vi "HighEnd-FPGA.vi"() -> ()   [LabVIEW 2016]
uses:
  Aperture Readback.ctl
  Faraday Cup Readback.ctl
  Glassman Readback.ctl
  Glassman Control.ctl
  <vilib>/LabVIEW Targets/FPGA/cRIO/shared/nicrio_ModuleControls/nicrio_cRIO-9871_BaudRateEnum.ctl
  <vilib>/LabVIEW Targets/FPGA/cRIO/shared/nicrio_ModuleControls/nicrio_cRIO-9871_DataBitsEnum.ctl
  <vilib>/LabVIEW Targets/FPGA/cRIO/shared/nicrio_ModuleControls/nicrio_cRIO-9871_ParityEnum.ctl
  <vilib>/LabVIEW Targets/FPGA/cRIO/shared/nicrio_ModuleControls/nicrio_cRIO-9871_StopBitsEnum.ctl
  <vilib>/Platform/TimedLoop/XDataNode/timing_clust.ctl
  <vilib>/Platform/TimedLoop/XDataNode/nitl_modes.ctl
  <vilib>/Platform/TimedLoop/XDataNode/wakeup.ctl
  <vilib>/rvi/FXPMathLib/basic elements/FxpIntAccumulator/subVIs/nifxpmath_IntAccumulator_SimConfig.ctl
  Gate Valve Readback.ctl
  <vilib>/rvi/Emulation/niFpgaGetClockAttributes.vi
  <vilib>/rvi/Emulation/niFpgaSctlEmulationGetInTimedLoop.vi
  <vilib>/rvi/Emulation/niFpgaEmulationReportErrorSimple.vi
  <vilib>/rvi/eio/common/nirviEmuTemplateMethod_errors.vi
  <vilib>/rvi/Emulation/niFpgaCriticalErrorInLSC.vi
  <vilib>/rvi/Analysis/common/codeGenErrors/XNode/niFpgaXNodeCodeGenErrorHandle.vi
  <vilib>/rvi/FXPMathLib/basic elements/FxpIntAccumulator/simVIs/DllFxpIntAccumulator_sub.vi
  <vilib>/rvi/eio/common/nirviEmuTemplatePropertySet_errors.vi
  <vilib>/eio/EIONode/EIONode.xnode
  <vilib>/rvi/Analysis/measure/dc-rms/XNode/niFpgaDC-RMS.xnode
  <vilib>/Platform/TimedLoop/XDataNode/XDataNode.xnode
  <vilib>/rvi/FXPMathLib/basic elements/FxpIntAccumulator/XNode/nifxpmath_IntAccumulator.xnode
  <vilib>/rvi/FXPMathLib/FxpMul/XNode/nifxpmath_Multiplier.xnode
  <vilib>/eio/EIOPropertyNode/EIOPropertyNode.xnode
  <vilib>/eio/EIOMethodNode/EIOMethodNode.xnode
  <vilib>/Platform/TimedLoop/XDataNode/XDNodeRunTimeDep.lvlib
  <vilib>/rvi/FXPMathLib/sim/FxpSim.dll
  <vilib>/rvi/eio/common/nirviEmuTemplatePropertyGet_errors.vi
  <vilib>/rvi/eio/common/nirviEmuTemplatePropertyGet_noerrors.vi
  <vilib>/rvi/eio/common/nirviEmuTemplatePropertySet_noerrors.vi
panel:
  out "HV control loop error":errorcluster
  in  "ES Quad A V set":T1
  in  "Y1- Steerer V set":T1
  in  "ES Quad B V set":T1
  in  "Y2- Steerer V set":T1
  in  "Y2+ Steerer V set":T1
  in  "Y1+ Steerer V set":T1
  in  "X- Steerer V set":T1
  in  "X+ Steerer V set":T1
  out "ES Quad HV readback loop error":errorcluster
  out "ES Quad B- readback":T2
  out "ES Quad B+ readback":T2
  out "ES Quad A- readback":T2
  out "ES Quad A+ readback":T2
  out "Steerer HV readback loop error":errorcluster
  out "Y2- Steerer readback":T2
  out "Y2+ Steerer readback":T2
  out "Y1- Steerer readback":T2
  out "Y1+ Steerer readback":T2
  out "X- Steerer readback":T2
  out "X+ Steerer readback":T2
  out "Analyzer Object Ion Gauge 2":u8[](array[numeric])
  out "Analyzer Object Convectron 2":u8[](array[numeric])
  out "Analyzer Object Convectron 1":u8[](array[numeric])
  out "Analyzer Object Ion Gauge 1":u8[](array[numeric])
  out "Analyzer Obj Vac Gauge error":errorcluster
  out "Tank Exit Ion Gauge 2":u8[](array[numeric])
  out "Tank Exit Convectron 2":u8[](array[numeric])
  out "Tank Exit Convectron 1":u8[](array[numeric])
  out "Tank Exit Ion Gauge 1":u8[](array[numeric])
  out "Tank Exit Vac Gauge error":errorcluster
  out "Beamline Fast GV Position":T3
  in  "Tank Exit FC Actuator":bool
  out "Tank Exit FC Position":T4
  out "Beamline GV Position":T4
  out "Cryo Pump GV Position":T3
  out "Turbo GV Position":T3
  out "Actuator loop error":errorcluster
  in  "Beamline GV Actuator":bool
  in  "Cryo Pump GV Actuator":bool
  in  "Turbo GV actuator":bool
  in  "Beamline Fast GV actuator":bool
  out "Tank Exit Vac Interlock":bool
  out "High End Waist Vac Interlock":bool
  in  "Analyzer Image Vac Interlock":bool
  in  "Tank Exit interlock bypass":bool
  in  "High End waist interlock bypass":bool
  out "GV Interlock loop error 2":errorcluster
  in  "RT error":bool
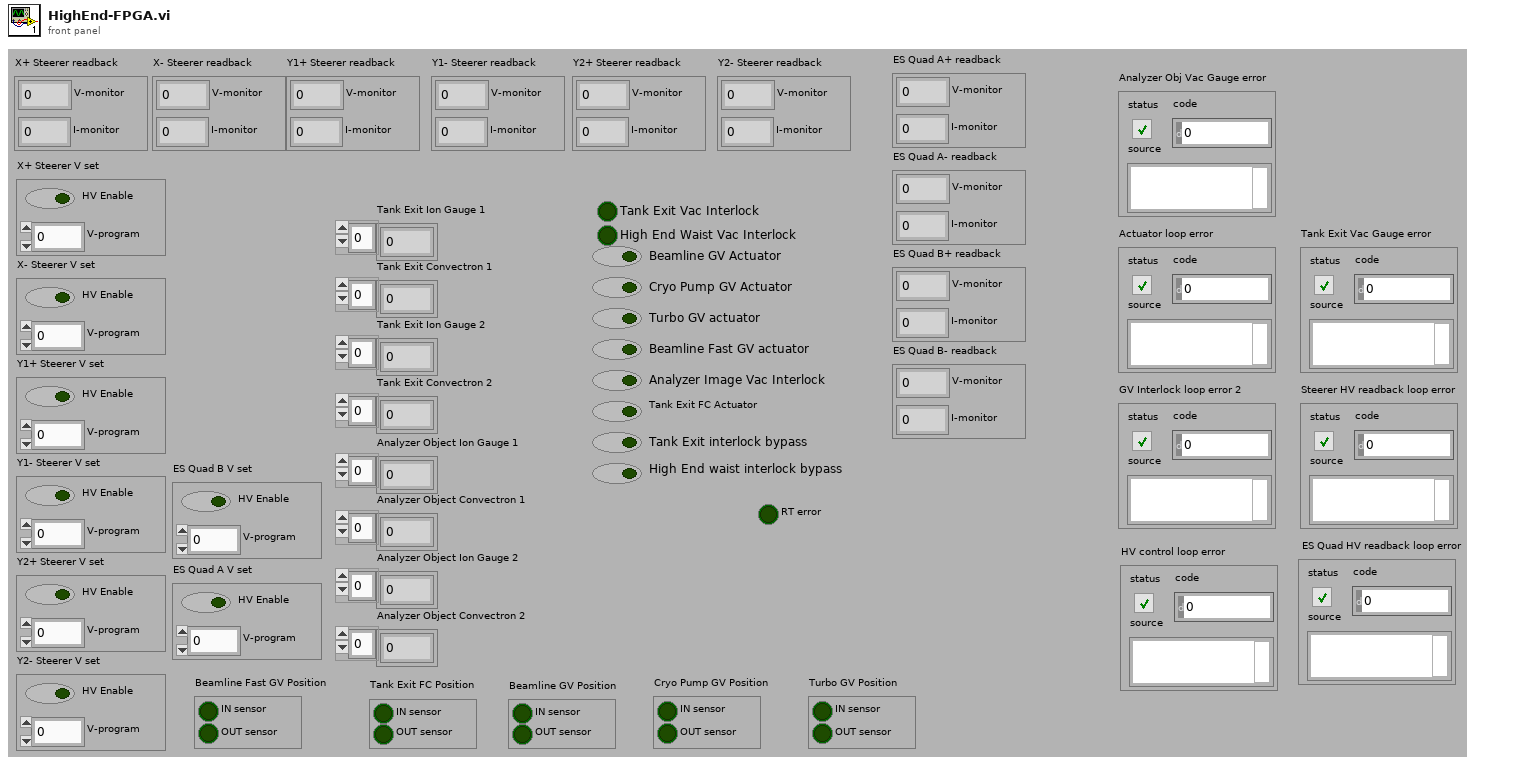
[diagram p1: front panel]
types:
  T1 = typedef "Glassman Control.ctl" = cluster{"V-program":fxp<+/-,20,5>, "HV Enable":bool}
  T2 = typedef "Glassman Readback.ctl" = cluster{"I-monitor":fxp<+/-,26,5>, "V-monitor":fxp<+/-,26,7>}
  T3 = typedef "Aperture Readback.ctl" = cluster{"IN sensor":bool, "OUT sensor":bool}
  T4 = typedef "Faraday Cup Readback.ctl" = cluster{"IN sensor":bool, "OUT sensor":bool}
  T5 = typedef "nicrio_cRIO-9871_StopBitsEnum.ctl" = enum8{"1", "1.5", "2"}
  T6 = typedef "nicrio_cRIO-9871_ParityEnum.ctl" = enum8{"None", "Odd", "Even", "Mark", "Space"}
  T7 = typedef "nicrio_cRIO-9871_DataBitsEnum.ctl" = enum8{"5", "6", "7", "8"}
  T8 = typedef "nicrio_cRIO-9871_BaudRateEnum.ctl" = enum16{"75 bps", "110 bps", "134 bps", "150 bps", "300 bps", "600 bps", "1200 bps", "1800 bps", "2400 bps", "4800 bps", "7200 bps", "9600 bps", "14.4 kbps", "19.2 kbps", "28.8 kbps", "38.4 kbps", "57.6 kbps", "115.2 kbps", "230.4 kbps", "460.8 kbps", "921.6 kbps"}
  T9 = typedef "Gate Valve Readback.ctl" = cluster{"OPEN sensor":bool, "Closed sensor":bool}
  T10 = typedef "XDNodeRunTimeDep.lvlib/timing_clust.ctl" = cluster{"Expected End [f-1]":u64, "Actual End [f-1]":u64, "Finished Late? [f-1]":bool, "Expected End [i-1]":u64, "Actual End [i-1]":u64, "Finished Late? [i-1]":bool, "Expected Start [i]":u64, "Actual Start [i]":u64, "Expected Start [f]":u64, "Actual Start [f]":u64, "Source Name":string, "Structure Name":string, "Period":i64, "Deadline":i64, "Offset":i64, "Start":i64, "Priority":i32, "Timeout":i32, "Mode":T11, "Wakeup Reason":T12, "Error":errorcluster, "Source Type":string, "Secondary Source Type":string, "Global End Time":u64, "Global Start Time":u64, "Frame Duration":u64, "Iteration Duration":u64, "Assigned CPU":i32, "I/O Scan Engine Mode":u32}
  T11 = typedef "XDNodeRunTimeDep.lvlib/nitl_modes.ctl" = enum32{"No Change", "Process missed periods, maintain original phase", "Discard missed periods, maintain original phase", "Process missed periods, ignore original phase", "Discard missed periods, ignore original phase"}
  T12 = typedef "XDNodeRunTimeDep.lvlib/wakeup.ctl" = enum32{"Normal", "Aborted", "Asynchronous wakeup", "Timing source error", "Timed loop error", "Timeout"}
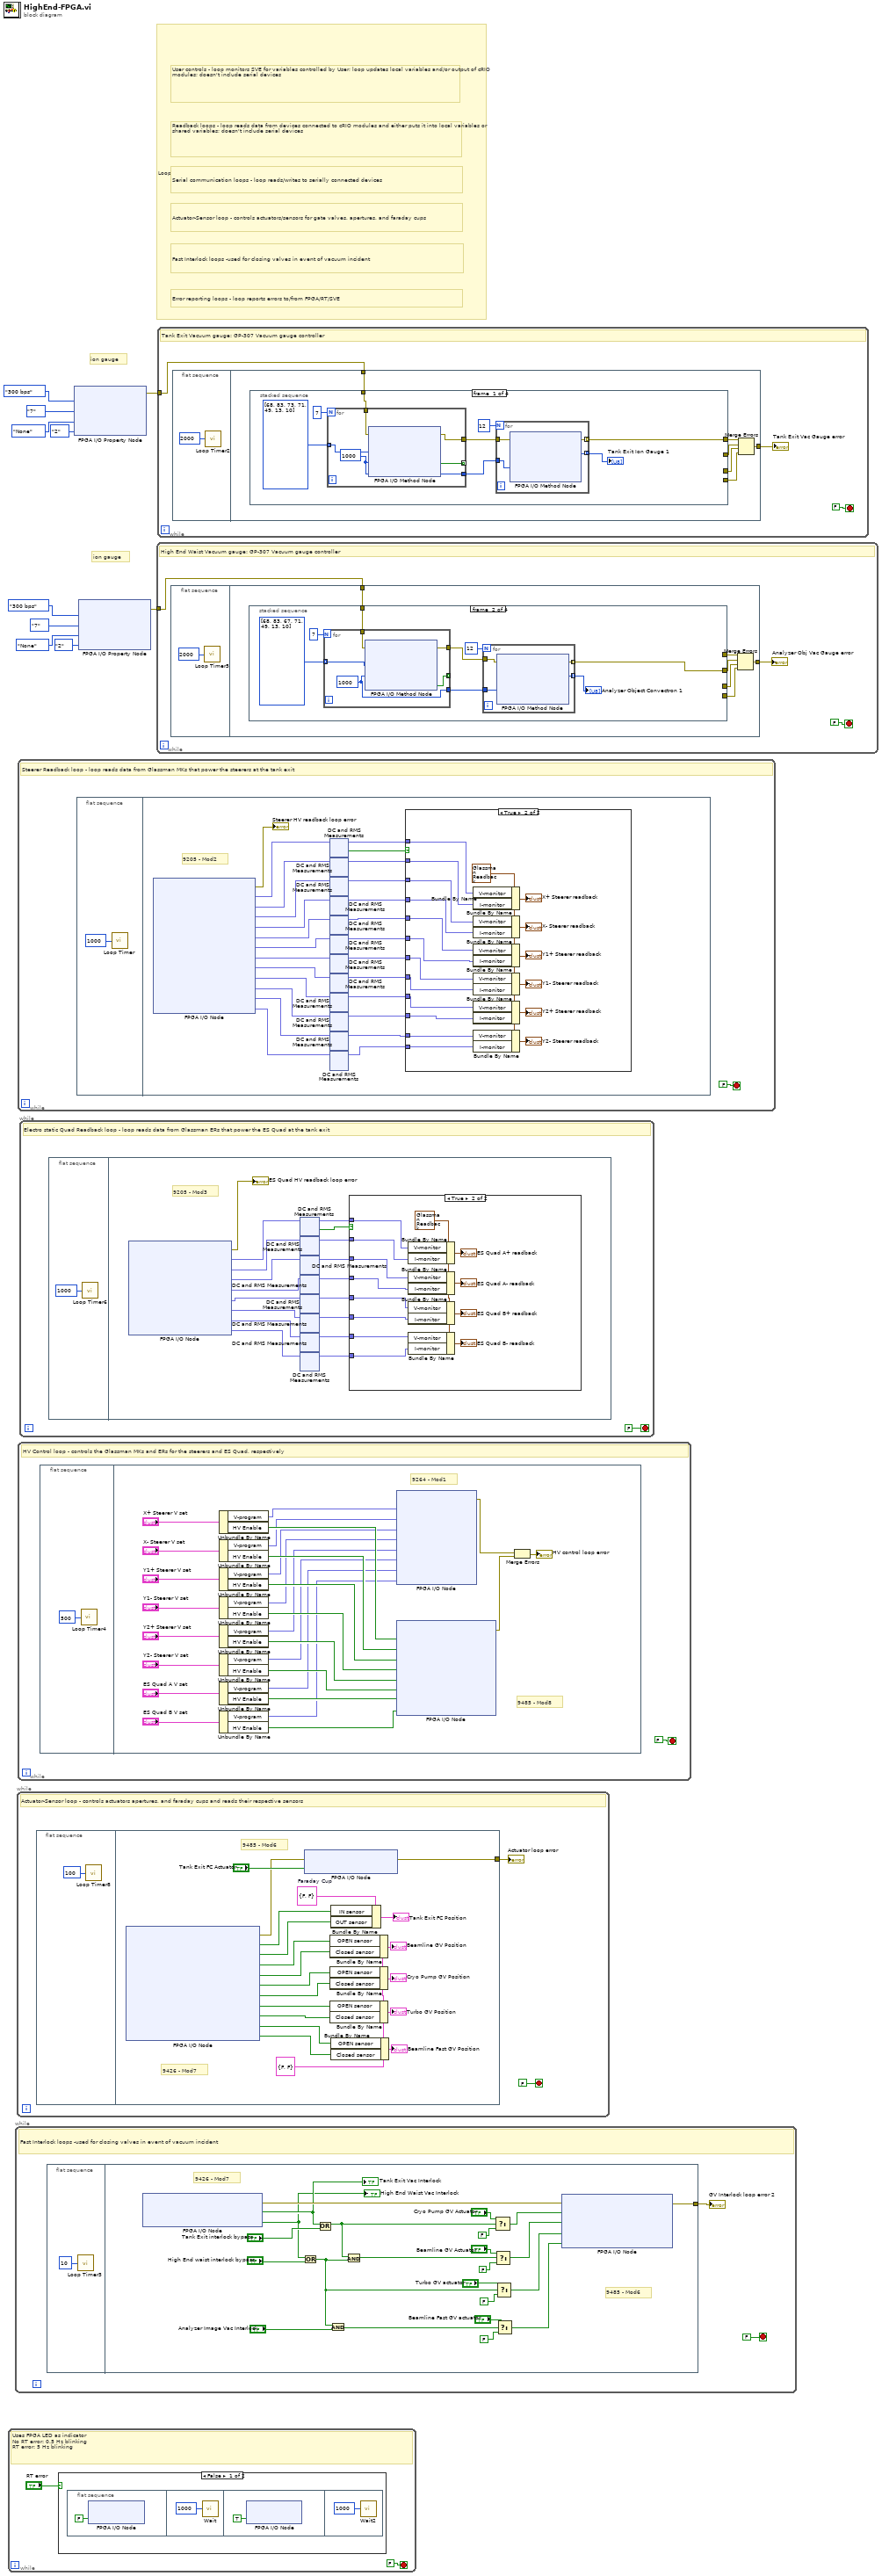
[diagram p0: block diagram]
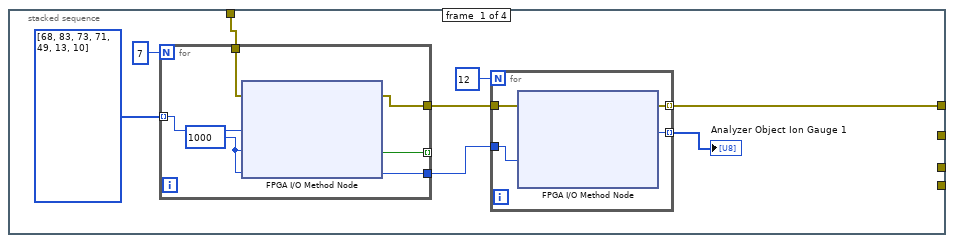
[diagram p3: hidden frame]
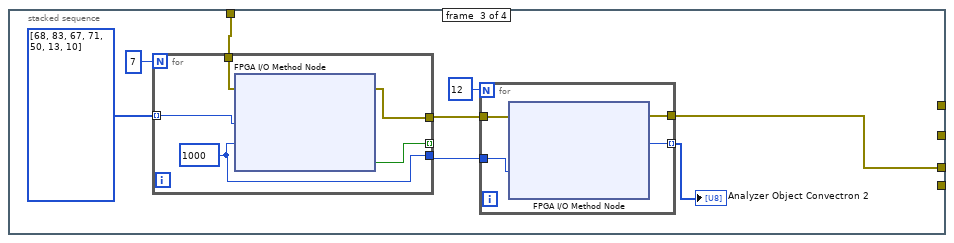
[diagram p4: hidden frame]
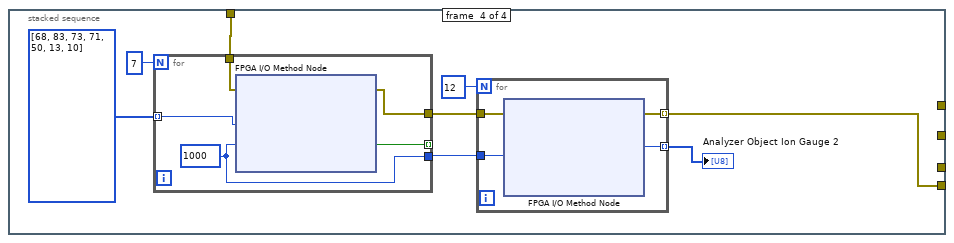
[diagram p5: hidden frame]
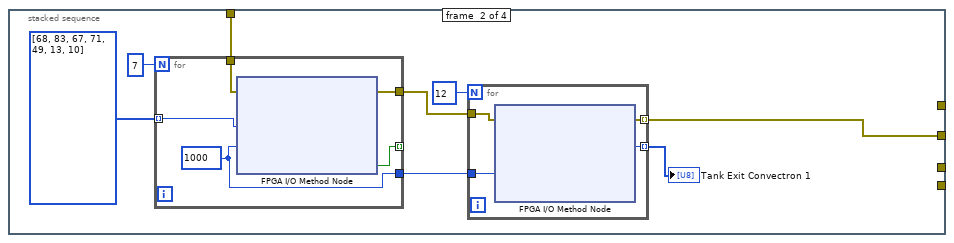
[diagram p6: hidden frame]
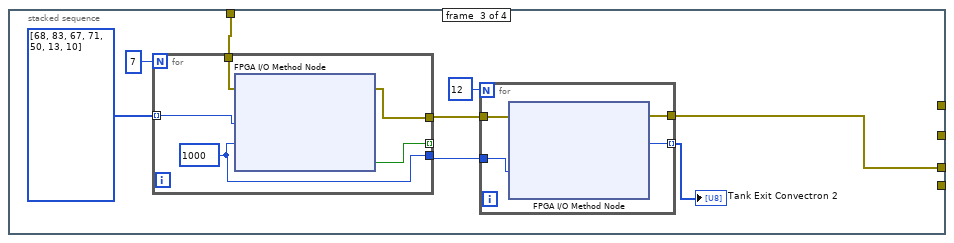
[diagram p7: hidden frame]
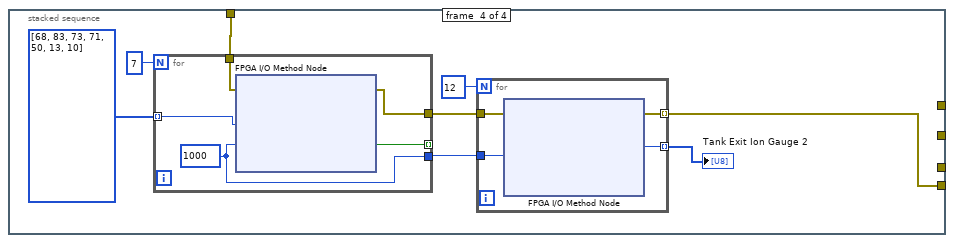
[diagram p8: hidden frame]
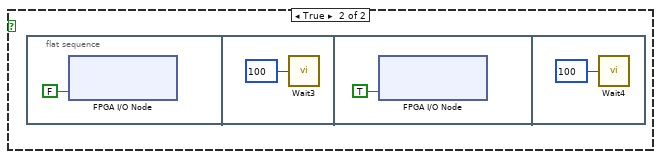
[diagram p9: hidden frame]
diagram:
  # "ion gauge"
  # "ion gauge"
  # "Actuator-Sensor loop - controls actuators/sensors for gate valves, apertures, and faraday cups"
  # "Fast Interlock loops -used for closing valves in event of vacuum incident"
  # "Error reporting loops - loop reports errors to/from FPGA/RT/SVE"
  # "Serial communication loops - loop reads/writes to serially connected devices"
  # "Readback loops - loop reads data from devices connected to cRIO modules and either puts it into local variables or shared variables; doesn't include serial devices"
  # "User controls - loop monitors SVE for variables controlled by User; loop updates local variables and/or output of cRIO modules; doesn't include serial devices"
  # "Loop legend - loops are color coded by responsibility"
  n1 = while {
    stop <- FALSE stop-if-true
    # "Uses FPGA LED as indicator\nNo RT error: 0.5 Hz blinking\nRT error: 5 Hz blinking"
    n2 = case shown="False" "RT error" {
      frame False {
        n3 = flat-sequence {
          frame #0 {
            n4 = xnode "FPGA I/O Node"("FPGA LED"=FALSE) -> ()  [unwired: 1 in, 1 out]
          }
          frame #1 {
            n5 = call "Wait"("Count(mSec)"=u16 1000) -> ()  [unwired: 1 out]
          }
          frame #2 {
            n6 = xnode "FPGA I/O Node"("FPGA LED"=TRUE) -> ()  [unwired: 1 in, 1 out]
          }
          frame #3 {
            n7 = call "Wait2"("Count(mSec)"=u16 1000) -> ()  [unwired: 1 out]
          }
        }
      }
      frame True {
        n8 = flat-sequence {
          frame #0 {
            n9 = xnode "FPGA I/O Node"("FPGA LED"=FALSE) -> ()  [unwired: 1 in, 1 out]
          }
          frame #1 {
            n10 = call "Wait3"("Count(mSec)"=u16 100) -> ()  [unwired: 1 out]
          }
          frame #2 {
            n11 = xnode "FPGA I/O Node"("FPGA LED"=TRUE) -> ()  [unwired: 1 in, 1 out]
          }
          frame #3 {
            n12 = call "Wait4"("Count(mSec)"=u16 100) -> ()  [unwired: 1 out]
          }
        }
      }
    }
  }
  n13 = while {
    stop <- FALSE stop-if-true
    # "Fast Interlock loops -used for closing valves in event of vacuum incident"
    n14 = flat-sequence {
      tunnel: [w35] -> w21
      frame #0 {
        n15 = call "Loop Timer3"("Count(uSec)"=u32 10) -> ()  [unwired: 1 out]
      }
      frame #1 {
        # "9485 - Mod6"
        # "9426 - Mod7"
        n16 = xnode "FPGA I/O Node"() -> ("error out"=w46:errorcluster, "Tank Exit Vac Interlock"=w34:bool, "High End Waist Vac Interlock"=w32:bool)  [unwired: 3 in, 2 out]
        "Tank Exit Vac Interlock" <- w34
        "High End Waist Vac Interlock" <- w32
        n17 = Or(x=w32, y="High End waist interlock bypass") -> (x .or. y?=w25:bool)
        n18 = Or(x=w34, y="Tank Exit interlock bypass") -> (x .or. y?=w24:bool)
        n19 = And(x=w25, y="Analyzer Image Vac Interlock") -> (x .and. y?=w30:bool)
        n20 = And(x=w24, y=w25) -> (x .and. y?=w26:bool)
        n21 = Select(t="Cryo Pump GV Actuator", s=w24, f=FALSE) -> (s? t:f=w36:bool)
        n22 = Select(t="Beamline GV Actuator", s=w26, f=FALSE) -> (s? t:f=w38:bool)
        n23 = Select(t="Turbo GV actuator", s=w25, f=FALSE) -> (s? t:f=w41:bool)
        n24 = Select(t="Beamline Fast GV actuator", s=w30, f=FALSE) -> (s? t:f=w44:bool)
        n25 = xnode "FPGA I/O Node"("error in"=w46, "Cryo Pump GV actuator"=w36, "Beamline GV actuator"=w38, "Turbo GV actuator"=w41, "Beamline Fast GV actuator"=w44) -> ("error out"=w35:errorcluster)  [unwired: 4 in, 4 out]
      }
    }
    "GV Interlock loop error 2" <- w21
  }
  n26 = while {
    stop <- FALSE stop-if-true
    # "Actuator-Sensor loop - controls actuators apertures, and faraday cups and reads their respective sensors"
    n27 = flat-sequence {
      tunnel: [w68] -> w47
      frame #0 {
        n28 = call "Loop Timer8"("Count(mSec)"=u32 100 ("Count(uSec)")) -> ()  [unwired: 1 out]
      }
      frame #1 {
        w52 = T9 {"OPEN sensor"=FALSE, "Closed sensor"=FALSE} ("Gate Valve")
        w64 = T4 {"IN sensor"=FALSE, "OUT sensor"=FALSE}  # Faraday Cup
        # "9485 - Mod6"
        # "9426 - Mod7"
        n29 = xnode "FPGA I/O Node"() -> ("error out"=w67:errorcluster, "Tank Exit FC IN sensor"=w66:bool, "Tank Exit FC OUT sensor"=w65:bool, "Beamline GV OPEN sensor"=w59:bool, "Beamline GV CLOSED sensor"=w58:bool, "Cryo Pump GV OPEN sensor"=w57:bool, "Cryo Pump GV CLOSED sensor"=w56:bool, "Turbo GV OPEN sensor"=w55:bool, "Turbo GV CLOSED sensor"=w54:bool, "Beamline Fast GV OPEN sensor"=w51:bool, "Beamline Fast GV CLOSED sensor"=w50:bool)  [unwired: 11 in, 10 out]
        n30 = xnode "FPGA I/O Node"("error in"=w67, "Tank Exit FC actuator"="Tank Exit FC Actuator") -> ("error out"=w68:errorcluster)  [unwired: 1 in, 1 out]
        n31 = Bundle By Name(cluster=w52, "OPEN sensor"=w59, "Closed sensor"=w58) -> (→"Beamline GV Position":T9)
        n32 = Bundle By Name(cluster=w52, "OPEN sensor"=w57, "Closed sensor"=w56) -> (→"Cryo Pump GV Position":T9)
        n33 = Bundle By Name(cluster=w52, "OPEN sensor"=w55, "Closed sensor"=w54) -> (→"Turbo GV Position":T9)
        n34 = Bundle By Name(cluster=w64, "IN sensor"=w66, "OUT sensor"=w65) -> (→"Tank Exit FC Position":T4)
        n35 = Bundle By Name(cluster=w52, "OPEN sensor"=w51, "Closed sensor"=w50) -> (→"Beamline Fast GV Position":T9)
      }
    }
    "Actuator loop error" <- w47
  }
  n36 = while {
    stop <- FALSE stop-if-true
    # "Steerer Readback loop - loop reads data from Glassman MKs that power the steerers at the tank exit"
    n37 = flat-sequence {
      frame #0 {
        n38 = call "Loop Timer"("Count(Ticks)"=u32 1000) -> ()  [unwired: 1 out]
      }
      frame #1 {
        # "9205 - Mod2"
        n39 = xnode "FPGA I/O Node"() -> ("error out"=→"Steerer HV readback loop error":errorcluster, "X+ Steerer V readback"=w96:fxp<+/-,26,5>, "X+ Steerer I readback"=w94:fxp<+/-,26,5>, "X- Steerer V readback"=w92:fxp<+/-,26,5>, "X- Steerer I readback"=w90:fxp<+/-,26,5>, "Y1+ Steerer V readback"=w88:fxp<+/-,26,5>, "Y1+ Steerer I readback"=w86:fxp<+/-,26,5>, "Y1- Steerer V readback"=w84:fxp<+/-,26,5>, "Y1- Steerer I readback"=w82:fxp<+/-,26,5>, "Y2+ Steerer V readback"=w80:fxp<+/-,26,5>, "Y2+ Steerer I readback"=w78:fxp<+/-,26,5>, "Y2- Steerer V readback"=w76:fxp<+/-,26,5>, "Y2- Steerer I readback"=w73:fxp<+/-,26,5>)  [unwired: 13 in, 12 out]
        n40 = xnode "DC and RMS Measurements"("input data"=w96) -> ("DC"=w95:fxp<+/-,26,5>, "output valid"=w97:bool)  [unwired: 1 in]
        n41 = xnode "DC and RMS Measurements"("input data"=w94) -> ("DC"=w93:fxp<+/-,26,5>)  [unwired: 1 in, 1 out]
        n42 = xnode "DC and RMS Measurements"("input data"=w92) -> ("DC"=w91:fxp<+/-,26,5>)  [unwired: 1 in, 1 out]
        n43 = xnode "DC and RMS Measurements"("input data"=w90) -> ("DC"=w89:fxp<+/-,26,5>)  [unwired: 1 in, 1 out]
        n44 = xnode "DC and RMS Measurements"("input data"=w88) -> ("DC"=w87:fxp<+/-,26,5>)  [unwired: 1 in, 1 out]
        n45 = xnode "DC and RMS Measurements"("input data"=w86) -> ("DC"=w85:fxp<+/-,26,5>)  [unwired: 1 in, 1 out]
        n46 = xnode "DC and RMS Measurements"("input data"=w84) -> ("DC"=w83:fxp<+/-,26,5>)  [unwired: 1 in, 1 out]
        n47 = xnode "DC and RMS Measurements"("input data"=w82) -> ("DC"=w81:fxp<+/-,26,5>)  [unwired: 1 in, 1 out]
        n48 = xnode "DC and RMS Measurements"("input data"=w80) -> ("DC"=w79:fxp<+/-,26,5>)  [unwired: 1 in, 1 out]
        n49 = xnode "DC and RMS Measurements"("input data"=w78) -> ("DC"=w77:fxp<+/-,26,5>)  [unwired: 1 in, 1 out]
        n50 = xnode "DC and RMS Measurements"("input data"=w76) -> ("DC"=w75:fxp<+/-,26,5>)  [unwired: 1 in, 1 out]
        n51 = xnode "DC and RMS Measurements"("input data"=w73) -> ("DC"=w74:fxp<+/-,26,5>)  [unwired: 1 in, 1 out]
        n52 = case shown="True" w97 {
          tunnel: w95 -> [_ w196]
          tunnel: w93 -> [_ w195]
          tunnel: w91 -> [_ w194]
          tunnel: w89 -> [_ w193]
          tunnel: w87 -> [_ w192]
          tunnel: w85 -> [_ w191]
          tunnel: w83 -> [_ w190]
          tunnel: w81 -> [_ w189]
          tunnel: w79 -> [_ w188]
          tunnel: w77 -> [_ w187]
          tunnel: w75 -> [_ w186]
          tunnel: w74 -> [_ w185]
          frame False {
          }
          frame True {
            w178 = T2 {"I-monitor"=0.0, "V-monitor"=0.0} ("Glassman Readback")
            n53 = Bundle By Name(cluster=w178, "V-monitor"=w196, "I-monitor"=w195) -> (→"X+ Steerer readback":T2)
            n54 = Bundle By Name(cluster=w178, "V-monitor"=w194, "I-monitor"=w193) -> (→"X- Steerer readback":T2)
            n55 = Bundle By Name(cluster=w178, "V-monitor"=w192, "I-monitor"=w191) -> (→"Y1+ Steerer readback":T2)
            n56 = Bundle By Name(cluster=w178, "V-monitor"=w190, "I-monitor"=w189) -> (→"Y1- Steerer readback":T2)
            n57 = Bundle By Name(cluster=w178, "V-monitor"=w188, "I-monitor"=w187) -> (→"Y2+ Steerer readback":T2)
            n58 = Bundle By Name(cluster=w178, "V-monitor"=w186, "I-monitor"=w185) -> (→"Y2- Steerer readback":T2)
          }
        }
      }
    }
  }
  n59 = while {
    stop <- FALSE stop-if-true
    # "HV Control loop - controls the Glassman MKs and ERs for the steerers and ES Quad, respectively"
    n60 = flat-sequence {
      frame #0 {
        n61 = call "Loop Timer4"("Count(uSec)"=u32 500 ("Count(Ticks)")) -> ()  [unwired: 1 out]
      }
      frame #1 {
        # "9485 - Mod8"
        # "9264 - Mod1"
        n62 = Unbundle By Name("X+ Steerer V set") -> ("V-program"=w1082:fxp<+/-,20,5>, "HV Enable"=w1090:bool)
        n63 = Unbundle By Name("X- Steerer V set") -> ("V-program"=w1083:fxp<+/-,20,5>, "HV Enable"=w1091:bool)
        n64 = Unbundle By Name("Y1+ Steerer V set") -> ("V-program"=w1084:fxp<+/-,20,5>, "HV Enable"=w1092:bool)
        n65 = Unbundle By Name("Y1- Steerer V set") -> ("V-program"=w1085:fxp<+/-,20,5>, "HV Enable"=w1093:bool)
        n66 = Unbundle By Name("Y2+ Steerer V set") -> ("V-program"=w1086:fxp<+/-,20,5>, "HV Enable"=w1094:bool)
        n67 = Unbundle By Name("Y2- Steerer V set") -> ("V-program"=w1087:fxp<+/-,20,5>, "HV Enable"=w1095:bool)
        n68 = Unbundle By Name("ES Quad A V set") -> ("V-program"=w1088:fxp<+/-,20,5>, "HV Enable"=w1096:bool)
        n69 = Unbundle By Name("ES Quad B V set") -> ("V-program"=w1089:fxp<+/-,20,5>, "HV Enable"=w1097:bool)
        n70 = xnode "FPGA I/O Node"("X+ Steerer V set"=w1082, "X- Steerer V set"=w1083, "Y1+ Steerer V set"=w1084, "Y1- Steerer V set"=w1085, "Y2+ Steerer V set"=w1086, "Y2- Steerer V set"=w1087, "ES Quad A V set"=w1088, "ES Quad B V set"=w1089) -> ("error out"=w1081:errorcluster)  [unwired: 9 in, 8 out]
        n71 = xnode "FPGA I/O Node"("X+ Steerer HV Enable"=w1090, "X- Steerer HV Enable"=w1091, "Y1+ Steerer HV Enable"=w1092, "Y1- Steerer HV Enable"=w1093, "Y2+ Steerer HV Enable"=w1094, "Y2- Steerer HV Enable"=w1095, "ES Quad A HV Enable"=w1096, "ES Quad B HV Enable"=w1097) -> ("error out"=w1080:errorcluster)  [unwired: 9 in, 8 out]
        n72 = Merge Errors(w1081, w1080) -> (→"HV control loop error":errorcluster)
      }
    }
  }
  n73 = while {
    stop <- FALSE stop-if-true
    # "Electro static Quad Readback loop - loop reads data from Glassman ERs that power the ES Quad at the tank exit"
    n74 = flat-sequence {
      frame #0 {
        n75 = call "Loop Timer6"("Count(Ticks)"=u32 1000) -> ()  [unwired: 1 out]
      }
      frame #1 {
        # "9205 - Mod3"
        n76 = xnode "FPGA I/O Node"() -> ("error out"=→"ES Quad HV readback loop error":errorcluster, "ES Quad A+ V readback"=w1117:fxp<+/-,26,5>, "ES Quad A+ I readback"=w1116:fxp<+/-,26,5>, "ES Quad A- V readback"=w1115:fxp<+/-,26,5>, "ES Quad A- I readback"=w1114:fxp<+/-,26,5>, "ES Quad B+ V readback"=w1113:fxp<+/-,26,5>, "ES Quad B+ I readback"=w1112:fxp<+/-,26,5>, "ES Quad B- V readback"=w1111:fxp<+/-,26,5>, "ES Quad B- I readback"=w1110:fxp<+/-,26,5>)  [unwired: 9 in, 8 out]
        n77 = xnode "DC and RMS Measurements"("input data"=w1117) -> ("DC"=w1125:fxp<+/-,26,5>, "output valid"=w1109:bool)  [unwired: 1 in]
        n78 = xnode "DC and RMS Measurements"("input data"=w1116) -> ("DC"=w1124:fxp<+/-,26,5>)  [unwired: 1 in, 1 out]
        n79 = xnode "DC and RMS Measurements"("input data"=w1115) -> ("DC"=w1123:fxp<+/-,26,5>)  [unwired: 1 in, 1 out]
        n80 = xnode "DC and RMS Measurements"("input data"=w1114) -> ("DC"=w1122:fxp<+/-,26,5>)  [unwired: 1 in, 1 out]
        n81 = xnode "DC and RMS Measurements"("input data"=w1113) -> ("DC"=w1121:fxp<+/-,26,5>)  [unwired: 1 in, 1 out]
        n82 = xnode "DC and RMS Measurements"("input data"=w1112) -> ("DC"=w1120:fxp<+/-,26,5>)  [unwired: 1 in, 1 out]
        n83 = xnode "DC and RMS Measurements"("input data"=w1111) -> ("DC"=w1119:fxp<+/-,26,5>)  [unwired: 1 in, 1 out]
        n84 = xnode "DC and RMS Measurements"("input data"=w1110) -> ("DC"=w1118:fxp<+/-,26,5>)  [unwired: 1 in, 1 out]
        n85 = case shown="True" w1109 {
          tunnel: w1125 -> [_ w1138]
          tunnel: w1124 -> [_ w1137]
          tunnel: w1123 -> [_ w1136]
          tunnel: w1122 -> [_ w1135]
          tunnel: w1121 -> [_ w1134]
          tunnel: w1120 -> [_ w1133]
          tunnel: w1119 -> [_ w1132]
          tunnel: w1118 -> [_ w1131]
          frame False {
          }
          frame True {
            w1130 = T2 {"I-monitor"=0.0, "V-monitor"=0.0} ("Glassman Readback")
            n86 = Bundle By Name(cluster=w1130, "V-monitor"=w1138, "I-monitor"=w1137) -> (→"ES Quad A+ readback":T2)
            n87 = Bundle By Name(cluster=w1130, "V-monitor"=w1136, "I-monitor"=w1135) -> (→"ES Quad A- readback":T2)
            n88 = Bundle By Name(cluster=w1130, "V-monitor"=w1134, "I-monitor"=w1133) -> (→"ES Quad B+ readback":T2)
            n89 = Bundle By Name(cluster=w1130, "V-monitor"=w1132, "I-monitor"=w1131) -> (→"ES Quad B- readback":T2)
          }
        }
      }
    }
  }
  n90 = xnode "FPGA I/O Property Node"("Baud Rate"=nicrio_cRIO-9871_BaudRateEnum."300 bps", "Data Bits"=nicrio_cRIO-9871_DataBitsEnum."7", "Parity"=nicrio_cRIO-9871_ParityEnum."None", "Stop Bits"=nicrio_cRIO-9871_StopBitsEnum."2") -> ("error out"=w2:errorcluster)  [unwired: 2 in, 1 out]
  n91 = xnode "FPGA I/O Property Node"("Baud Rate"=nicrio_cRIO-9871_BaudRateEnum."300 bps", "Data Bits"=nicrio_cRIO-9871_DataBitsEnum."7", "Parity"=nicrio_cRIO-9871_ParityEnum."None", "Stop Bits"=nicrio_cRIO-9871_StopBitsEnum."2") -> ("error out"=w1:errorcluster)  [unwired: 2 in, 1 out]
  n92 = while {
    tunnel: w1 -> [w1780]
    stop <- FALSE stop-if-true
    # "High End Waist Vacuum gauge: GP-307 Vacuum gauge controller"
    n93 = flat-sequence {
      tunnel: w1780 -> [w1788]
      tunnel: [w1783] -> w1779
      frame #0 {
        n94 = call "Loop Timer5"("Count(mSec)"=u32 2000 ("Count(Ticks)")) -> ()  [unwired: 1 out]
      }
      frame #1 {
        n95 = stacked-sequence {
          tunnel: [_ _ w1825 _] -> w1785
          tunnel: [_ _ _ w1841] -> w1784
          tunnel: w1788 -> [w1791 w1808 w1823 w1840]
          tunnel: [w1789 _ _ _] -> w1787
          tunnel: [_ w1807 _ _] -> w1786
          frame #0 {
            n96 = for {
              N: 7 -> [_]
              tunnel: [w1805] -> w1792
              tunnel: [w1804] -> _ mode=indexing
              tunnel: u8[] [68, 83, 73, 71, 49, 13, 10] ("unsigned byte array") -> [w1803] mode=indexing
              tunnel: w1791 -> [w1802]
              tunnel: [w1801] -> w1790
              w1805 = 1000 ("Timeout (ms)")
              n97 = xnode "FPGA I/O Method Node"("error in"=w1802, "Data"=w1803, "Timeout (ms)"=w1805) -> ("error out"=w1801:errorcluster, "Timed Out"=w1804:bool)  [unwired: 1 in, 1 out]
            }
            n98 = for {
              N: 12 -> [_]
              tunnel: w1792 -> [w1800]
              tunnel: [w1799] -> w1793 mode=indexing
              tunnel: w1790 -> [w1798]
              tunnel: [w1797] -> w1789 mode=indexing
              n99 = xnode "FPGA I/O Method Node"("error in"=w1798, "Timeout (ms)"=w1800) -> ("error out"=w1797:errorcluster, "Data"=w1799:u8)  [unwired: 1 in, 2 out]
            }
            "Analyzer Object Ion Gauge 1" <- w1793
          }
          frame #1 {
            n100 = for {
              N: 7 -> [_]
              tunnel: [w1821] -> w1813
              tunnel: [w1820] -> _ mode=indexing
              tunnel: u8[] [68, 83, 67, 71, 49, 13, 10] ("unsigned byte array") -> [w1822] mode=indexing
              tunnel: w1808 -> [w1819]
              tunnel: [w1818] -> w1806
              w1821 = 1000 ("Timeout (ms)")
              n101 = xnode "FPGA I/O Method Node"("error in"=w1819, "Data"=w1822, "Timeout (ms)"=w1821) -> ("error out"=w1818:errorcluster, "Timed Out"=w1820:bool)  [unwired: 1 in, 1 out]
            }
            n102 = for {
              N: 12 -> [_]
              tunnel: w1813 -> [w1817]
              tunnel: [w1816] -> w1809 mode=indexing
              tunnel: w1806 -> [w1815]
              tunnel: [w1814] -> w1807 mode=indexing
              n103 = xnode "FPGA I/O Method Node"("error in"=w1815, "Timeout (ms)"=w1817) -> ("error out"=w1814:errorcluster, "Data"=w1816:u8)  [unwired: 1 in, 2 out]
            }
            "Analyzer Object Convectron 1" <- w1809
          }
          frame #2 {
            n104 = for {
              N: 7 -> [_]
              tunnel: [w1837] -> w1830
              tunnel: [w1838] -> _ mode=indexing
              tunnel: u8[] [68, 83, 67, 71, 50, 13, 10] ("unsigned byte array") -> [w1839] mode=indexing
              tunnel: [w1836] -> w1826
              tunnel: w1823 -> [w1835]
              w1837 = 1000 ("Timeout (ms)")
              n105 = xnode "FPGA I/O Method Node"("error in"=w1835, "Data"=w1839, "Timeout (ms)"=w1837) -> ("error out"=w1836:errorcluster, "Timed Out"=w1838:bool)  [unwired: 1 in, 1 out]
            }
            n106 = for {
              N: 12 -> [_]
              tunnel: w1830 -> [w1834]
              tunnel: [w1833] -> w1824 mode=indexing
              tunnel: w1826 -> [w1832]
              tunnel: [w1831] -> w1825
              n107 = xnode "FPGA I/O Method Node"("error in"=w1832, "Timeout (ms)"=w1834) -> ("error out"=w1831:errorcluster, "Data"=w1833:u8)  [unwired: 1 in, 2 out]
            }
            "Analyzer Object Convectron 2" <- w1824
          }
          frame #3 {
            n108 = for {
              N: 7 -> [_]
              tunnel: [w1854] -> w1847
              tunnel: [w1856] -> _ mode=indexing
              tunnel: u8[] [68, 83, 73, 71, 50, 13, 10] ("unsigned byte array") -> [w1855] mode=indexing
              tunnel: [w1853] -> w1842
              tunnel: w1840 -> [w1852]
              w1854 = 1000 ("Timeout (ms)")
              n109 = xnode "FPGA I/O Method Node"("error in"=w1852, "Data"=w1855, "Timeout (ms)"=w1854) -> ("error out"=w1853:errorcluster, "Timed Out"=w1856:bool)  [unwired: 1 in, 1 out]
            }
            n110 = for {
              N: 12 -> [_]
              tunnel: w1847 -> [w1851]
              tunnel: [w1850] -> w1843 mode=indexing
              tunnel: w1842 -> [w1849]
              tunnel: [w1848] -> w1841 mode=indexing
              n111 = xnode "FPGA I/O Method Node"("error in"=w1849, "Timeout (ms)"=w1851) -> ("error out"=w1848:errorcluster, "Data"=w1850:u8)  [unwired: 1 in, 2 out]
            }
            "Analyzer Object Ion Gauge 2" <- w1843
          }
        }
        n112 = Merge Errors(w1787, w1786, w1785, w1784) -> (w1783:errorcluster)
      }
    }
    "Analyzer Obj Vac Gauge error" <- w1779
  }
  n113 = while {
    tunnel: w2 -> [w1858]
    stop <- FALSE stop-if-true
    # "Tank Exit Vacuum gauge: GP-307 Vacuum gauge controller"
    n114 = flat-sequence {
      tunnel: w1858 -> [w1866]
      tunnel: [w1861] -> w1857
      frame #0 {
        n115 = call "Loop Timer2"("Count(mSec)"=u32 2000 ("Count(Ticks)")) -> ()  [unwired: 1 out]
      }
      frame #1 {
        n116 = stacked-sequence {
          tunnel: [_ _ w1903 _] -> w1863
          tunnel: [_ _ _ w1919] -> w1862
          tunnel: w1866 -> [w1869 w1886 w1901 w1918]
          tunnel: [w1867 _ _ _] -> w1865
          tunnel: [_ w1885 _ _] -> w1864
          frame #0 {
            n117 = for {
              N: 7 -> [_]
              tunnel: [w1883] -> w1870
              tunnel: [w1882] -> _ mode=indexing
              tunnel: u8[] [68, 83, 73, 71, 49, 13, 10] ("unsigned byte array") -> [w1881] mode=indexing
              tunnel: w1869 -> [w1880]
              tunnel: [w1879] -> w1868
              w1883 = 1000 ("Timeout (ms)")
              n118 = xnode "FPGA I/O Method Node"("error in"=w1880, "Data"=w1881, "Timeout (ms)"=w1883) -> ("error out"=w1879:errorcluster, "Timed Out"=w1882:bool)  [unwired: 1 in, 1 out]
            }
            n119 = for {
              N: 12 -> [_]
              tunnel: w1870 -> [w1878]
              tunnel: [w1877] -> w1871 mode=indexing
              tunnel: w1868 -> [w1876]
              tunnel: [w1875] -> w1867 mode=indexing
              n120 = xnode "FPGA I/O Method Node"("error in"=w1876, "Timeout (ms)"=w1878) -> ("error out"=w1875:errorcluster, "Data"=w1877:u8)  [unwired: 1 in, 2 out]
            }
            "Tank Exit Ion Gauge 1" <- w1871
          }
          frame #1 {
            n121 = for {
              N: 7 -> [_]
              tunnel: [w1899] -> w1891
              tunnel: [w1898] -> _ mode=indexing
              tunnel: u8[] [68, 83, 67, 71, 49, 13, 10] ("unsigned byte array") -> [w1900] mode=indexing
              tunnel: w1886 -> [w1897]
              tunnel: [w1896] -> w1884
              w1899 = 1000 ("Timeout (ms)")
              n122 = xnode "FPGA I/O Method Node"("error in"=w1897, "Data"=w1900, "Timeout (ms)"=w1899) -> ("error out"=w1896:errorcluster, "Timed Out"=w1898:bool)  [unwired: 1 in, 1 out]
            }
            n123 = for {
              N: 12 -> [_]
              tunnel: w1891 -> [w1895]
              tunnel: [w1894] -> w1887 mode=indexing
              tunnel: w1884 -> [w1893]
              tunnel: [w1892] -> w1885 mode=indexing
              n124 = xnode "FPGA I/O Method Node"("error in"=w1893, "Timeout (ms)"=w1895) -> ("error out"=w1892:errorcluster, "Data"=w1894:u8)  [unwired: 1 in, 2 out]
            }
            "Tank Exit Convectron 1" <- w1887
          }
          frame #2 {
            n125 = for {
              N: 7 -> [_]
              tunnel: [w1915] -> w1908
              tunnel: [w1916] -> _ mode=indexing
              tunnel: u8[] [68, 83, 67, 71, 50, 13, 10] ("unsigned byte array") -> [w1917] mode=indexing
              tunnel: [w1914] -> w1904
              tunnel: w1901 -> [w1913]
              w1915 = 1000 ("Timeout (ms)")
              n126 = xnode "FPGA I/O Method Node"("error in"=w1913, "Data"=w1917, "Timeout (ms)"=w1915) -> ("error out"=w1914:errorcluster, "Timed Out"=w1916:bool)  [unwired: 1 in, 1 out]
            }
            n127 = for {
              N: 12 -> [_]
              tunnel: w1908 -> [w1912]
              tunnel: [w1911] -> w1902 mode=indexing
              tunnel: w1904 -> [w1910]
              tunnel: [w1909] -> w1903
              n128 = xnode "FPGA I/O Method Node"("error in"=w1910, "Timeout (ms)"=w1912) -> ("error out"=w1909:errorcluster, "Data"=w1911:u8)  [unwired: 1 in, 2 out]
            }
            "Tank Exit Convectron 2" <- w1902
          }
          frame #3 {
            n129 = for {
              N: 7 -> [_]
              tunnel: [w1932] -> w1925
              tunnel: [w1934] -> _ mode=indexing
              tunnel: u8[] [68, 83, 73, 71, 50, 13, 10] ("unsigned byte array") -> [w1933] mode=indexing
              tunnel: [w1931] -> w1920
              tunnel: w1918 -> [w1930]
              w1932 = 1000 ("Timeout (ms)")
              n130 = xnode "FPGA I/O Method Node"("error in"=w1930, "Data"=w1933, "Timeout (ms)"=w1932) -> ("error out"=w1931:errorcluster, "Timed Out"=w1934:bool)  [unwired: 1 in, 1 out]
            }
            n131 = for {
              N: 12 -> [_]
              tunnel: w1925 -> [w1929]
              tunnel: [w1928] -> w1921 mode=indexing
              tunnel: w1920 -> [w1927]
              tunnel: [w1926] -> w1919 mode=indexing
              n132 = xnode "FPGA I/O Method Node"("error in"=w1927, "Timeout (ms)"=w1929) -> ("error out"=w1926:errorcluster, "Data"=w1928:u8)  [unwired: 1 in, 2 out]
            }
            "Tank Exit Ion Gauge 2" <- w1921
          }
        }
        n133 = Merge Errors(w1865, w1864, w1863, w1862) -> (w1861:errorcluster)
      }
    }
    "Tank Exit Vac Gauge error" <- w1857
  }
